vi "Position Open Mission Accept Button.vi"(8 "error in (no error)":errorcluster, 11 "Button Ref":refnum<vi>) -> (0 "error out":errorcluster)   [LabVIEW 2014]
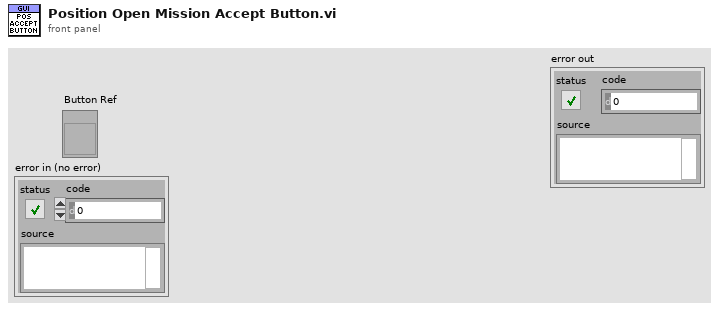
[diagram p1: front panel]
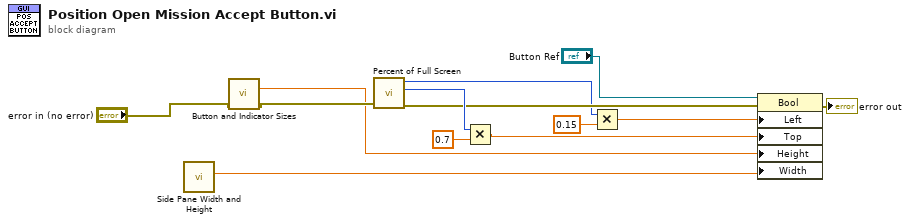
[diagram p0: block diagram]
diagram:
  n1 = call "Side Pane Width and Height.vi"() -> ("Width"=w8:dbl)  [unwired: 9 in, 2 out]
  n2 = call "Button and Indicator Sizes.vi"("error in (no error)"="error in (no error)") -> ("Button Height"=w9:dbl, "error out"=w11:errorcluster)  [unwired: 10 in, 3 out]
  n3 = call "Percent of Full Screen.vi"("error in (no error)"=w11) -> ("error out"=w5:errorcluster, "Bottom"=w7:i16, "Right"=w3:i16)  [unwired: 8 in]
  n4 = Multiply(x=w7, y=0.7) -> (x*y=w4:dbl)
  n5 = Multiply(x=w3, y=0.15) -> (x*y=w1:dbl)
  n6 = property class="Bool"(reference="Button Ref", error in=w5, "Left"=w1, "Top"=w4, "Height"=w9, "Width"=w8) -> (error out=→"error out":errorcluster)  [unwired: 1 out]
